vi "execute.vi"(8 "error in (no error)":errorcluster, 9 "B in":refnum<class "GenericComponent.lvclass">, 10 "A in":refnum<class "GenericComponent.lvclass">, 11 "AdapterMH111110ImagingModeToScanHead in":refnum<class "AdapterMH111110ImagingModeToScanHead.lvclass">) -> (0 "error out":errorcluster, 1 "B out":refnum<class "GenericComponent.lvclass">, 2 "A out":refnum<class "GenericComponent.lvclass">, 3 "AdapterMH111110ImagingModeToScanHead out":refnum<class "AdapterMH111110ImagingModeToScanHead.lvclass">)   [LabVIEW 2010, in "AdapterMH111110ImagingModeToScanHead.lvclass"]
uses:
  AdapterMH111110ImagingModeToScanHead.lvclass
  common/classes/GenericComponent/GenericComponent/GenericComponent.lvclass
  ImagingMode/ImagingModeDL090130Frame/ImagingModeDL090130Frame/translation_mode_enum.ctl
  ScanHead/ScanHeadMH100729FPGA/ScanHeadMH100729FPGA/ScanHeadMH100729FPGA.lvclass
  ImagingMode/ImagingModeDL090130Frame/ImagingModeDL090130Frame/settings_cluster.ctl
  ImagingMode/ImagingModeDL090130Frame/ImagingModeDL090130Frame/speed_constant_enum.ctl
  common/xcontrols/XIntensityCompensation/XIntensityCompensation/data.ctl
  ImagingMode/ImagingModeDL090130Frame/ImagingModeDL090130Frame/ImagingModeDL090130Frame.lvclass
  common/xcontrols/XIntensityCompensation/XIntensityCompensation/XIntensityCompensation.xctl
  ScanHead/ScanHeadMH100729FPGA/ScanHeadMH100729FPGA/settings_cluster.ctl
  ScanHead/ScanHeadMH100729FPGA/ScanHeadMH100729FPGA/intensity_adjustment_enum.ctl
  ScanHead/ScanHeadMH100729FPGA/ScanHeadMH100729FPGA/translation_mode_enum.ctl
  common/classes/ErrorController/ErrorController/class_data.vi
  common/classes/ErrorController/ErrorController/ErrorController.lvclass
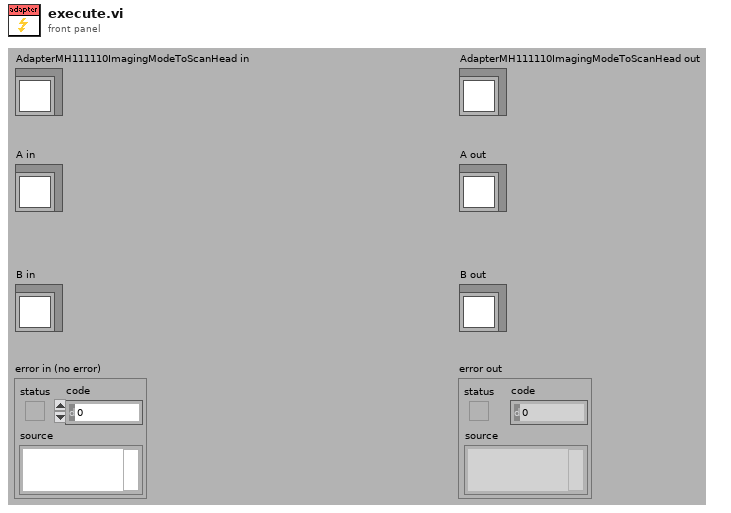
[diagram p1: front panel]
types:
  T1 = typedef "ImagingModeDL090130Frame.lvclass/translation_mode_enum.ctl" = enum16{"scanHead", "stage"}
  T2 = typedef "ImagingModeDL090130Frame.lvclass/settings_cluster.ctl" = cluster{"FrameSettings":cluster{"ResolutionX":i32, "ResolutionY":i32, "AspectRatioX":dbl, "AspectRatioY":dbl, "FrameScanRate":dbl[unit], "SpeedConstant":T3}, "StackSettings":cluster{"Frames":i32, "AveragingRepetitions":i32, "StepSize":dbl[unit], "ReturnToOrigin":bool, "TranslationMode":T1, "IntensityCompensationParameters":T4}}
  T3 = typedef "ImagingModeDL090130Frame.lvclass/speed_constant_enum.ctl" = enum16{"pixel dwell time", "line scan time", "frame rate"}
  T4 = typedef "XIntensityCompensation.xctl/data.ctl" = cluster{"A":dbl, "lambda":dbl[unit], "C":dbl}
  T5 = typedef "ScanHeadMH100729FPGA.lvclass/settings_cluster.ctl" = cluster{"Zoom":dbl, "Intensity":dbl, "AngleZ":dbl[unit], "AngleX":dbl[unit], "OffsetX":dbl[unit], "OffsetY":dbl[unit], "OffsetZ":dbl[unit], "ScatteringLength":dbl[unit], "intensity adjustment mode":T6, "translation mode":T7}
  T6 = typedef "ScanHeadMH100729FPGA.lvclass/intensity_adjustment_enum.ctl" = enum16{"manual", "look-up", "exponential"}
  T7 = typedef "ScanHeadMH100729FPGA.lvclass/translation_mode_enum.ctl" = enum16{"scan signal offset", "stage"}
  T8 = typedef "ImagingModeDL090130Frame.lvclass/control_refs.ctl" = cluster{"resolution controls":cluster{"x pixels":refnum<vi>, "y pixels":refnum<vi>, "ratio x factor":refnum<vi>, "ratio y factor":refnum<vi>}, "speed controls":cluster{"pixel dwell time":refnum<vi>, "line scan time":refnum<vi>, "frame rate":refnum<vi>, "keep constant":refnum<vi>}, "number of frames controls":cluster{"# of frames":refnum<vi>, "duration":refnum<vi>, "# of repetitions":refnum<vi>}, "current value indicators":cluster{"frame #":refnum<vi>, "repetition #":refnum<vi>, "offset":refnum<vi>}, "step controls":cluster{"step size":refnum<vi>, "return to origin?":refnum<vi>, "translation mode":refnum<vi>, "XIntensityCompensation":refnum<vi>}, "defineButton":refnum<vi>, "settings enforced?":refnum<vi>, "settings":refnum<vi>}
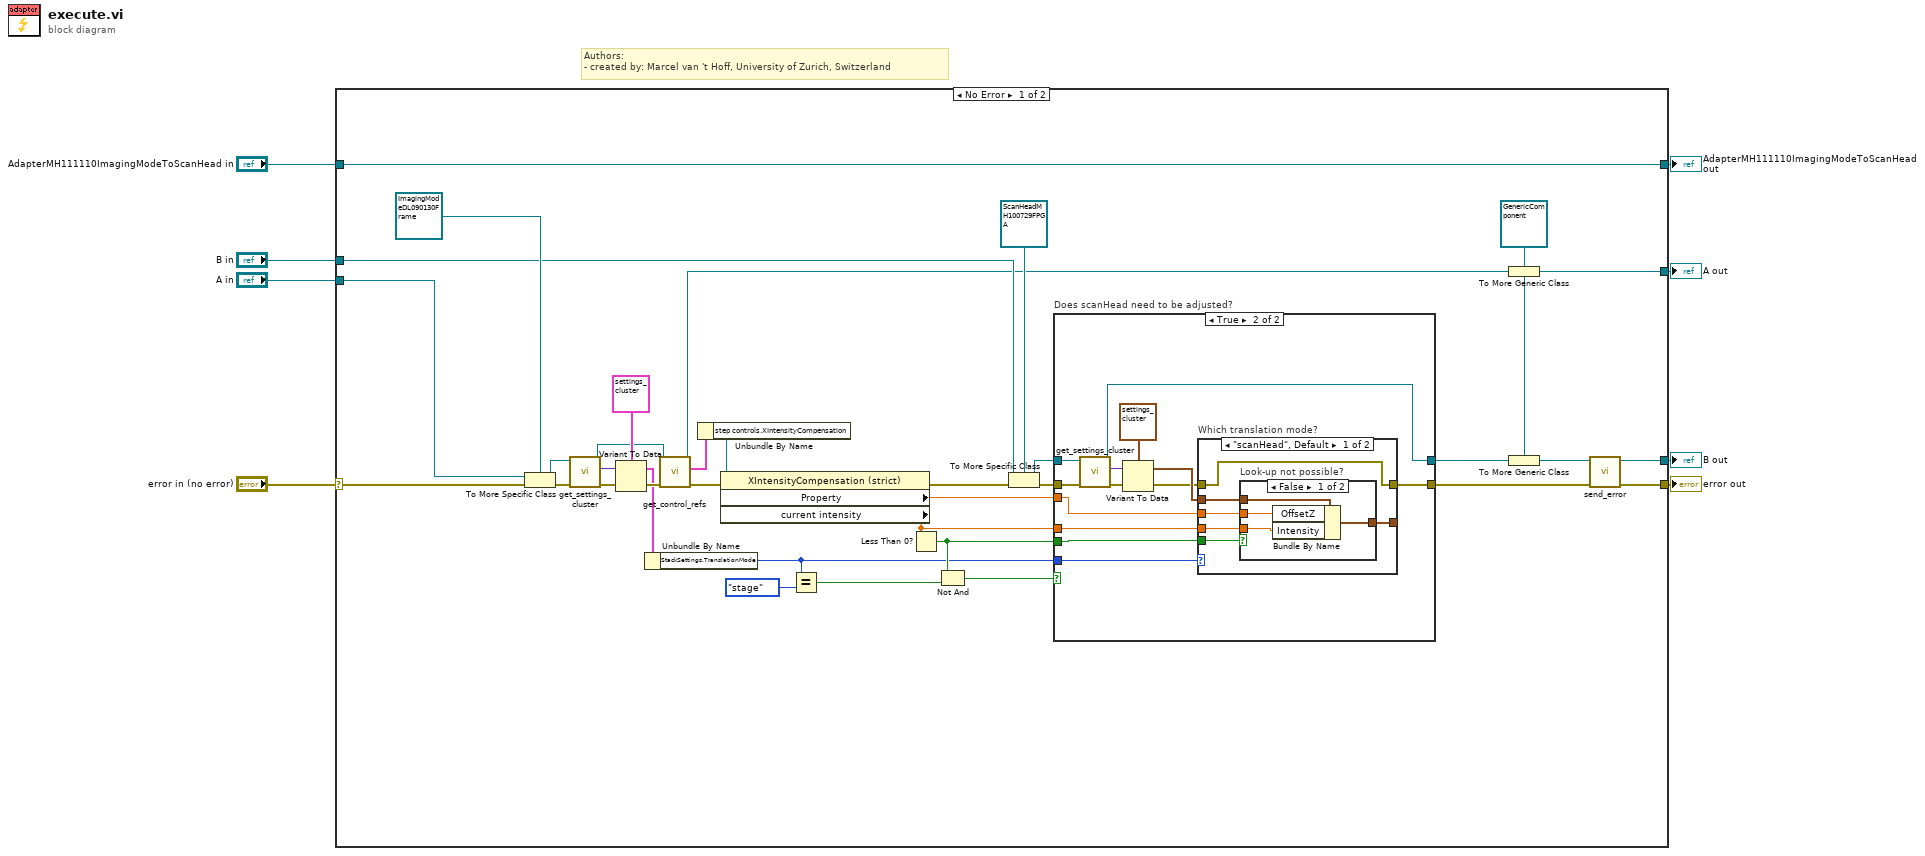
[diagram p0: block diagram]
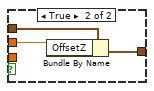
[diagram p3: hidden frame]
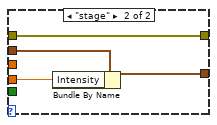
[diagram p4: hidden frame]
diagram:
  # "Authors: \n- created by: Marcel van 't Hoff, University of Zurich, Switzerland"
  n1 = case shown="No Error" "error in (no error)" {
    selector: "error in (no error)" -> [w39 w77]
    tunnel: [w10 w77] -> w7
    tunnel: [w42 w78] -> w6
    tunnel: "AdapterMH111110ImagingModeToScanHead in" -> [w42 w78]
    tunnel: "A in" -> [w41 w75]
    tunnel: "B in" -> [w27 w76]
    tunnel: [w14 w76] -> w2
    tunnel: [w11 w75] -> w1
    frame No Error {
      w13 = refnum<class "GenericComponent.lvclass"> refnum ("GenericComponent.lvclass")
      n2 = To More Specific Class(target class=refnum<class "ImagingModeDL090130Frame.lvclass"> refnum ("ImagingModeDL090130Frame.lvclass"), reference=w41, error in=w39) -> (specific class reference=w37:refnum<class "ImagingModeDL090130Frame.lvclass">, error out=w38:errorcluster)
      n3 = call-dynamic "get_settings_cluster.vi"("error in (no error)"=w38, "ImagingModeDL090130Frame in"=w37) -> ("error out"=w36:errorcluster, "settings cluster"=w35:variant, "ImagingModeDL090130Frame out"=w32:refnum<class "ImagingModeDL090130Frame.lvclass">)  [unwired: 7 in]
      n4 = Variant To Data(error in=w36, Variant=w35, type=T2 {"FrameSettings"={"ResolutionX"=0, "ResolutionY"=0, "AspectRatioX"=0.0, "AspectRatioY"=0.0, "FrameScanRate"=0.0, "SpeedConstant"=enum."pixel dwell time"}, "StackSettings"={"Frames"=0, "AveragingRepetitions"=0, "StepSize"=0.0, "ReturnToOrigin"=FALSE, "TranslationMode"=enum."scanHead", "IntensityCompensationParameters"={"A"=0.0, "lambda"=0.0, "C"=0.0}}} ("settings")) -> (error out=w33:errorcluster, data=w25:T2)
      n5 = Unbundle By Name(w25) -> ("StackSettings.TranslationMode"=w20:T1)
      n6 = call-dynamic "get_control_refs.vi"("error in (no error)"=w33, "ImagingModeDL090130Frame in"=w32) -> ("error out"=w30:errorcluster, "control refs"=w31:T8, "ImagingModeDL090130Frame out"=w12:refnum<class "ImagingModeDL090130Frame.lvclass">)  [unwired: 7 in]
      n7 = Unbundle By Name(w31) -> ("step controls.XIntensityCompensation"=w29:refnum<vi>)
      n8 = property class="XIntensityCompensation (strict)"(reference=w29, error in=w30) -> (error out=w28:errorcluster, "Property"=w19:dbl[unit], "current intensity"=w18:dbl)  [unwired: 1 out]
      n9 = Equal?(x=w20, y=translation_mode_enum."stage") -> (x = y?=w23:bool)
      n10 = Less Than 0?(x=w18) -> (x < 0?=w21:bool)
      n11 = Not And(1:w23, 2:w21) -> (0:w22:bool)
      n12 = To More Specific Class(target class=refnum<class "ScanHeadMH100729FPGA.lvclass"> refnum ("ScanHeadMH100729FPGA.lvclass"), reference=w27, error in=w28) -> (specific class reference=w16:refnum<class "ScanHeadMH100729FPGA.lvclass">, error out=w17:errorcluster)
      n13 = case "Does scanHead need to be adjusted?" shown="True" w22 {
        tunnel: w21 -> [_ w49]
        tunnel: w20 -> [_ w48]
        tunnel: w19 -> [_ w51]
        tunnel: w18 -> [_ w50]
        tunnel: w17 -> [w43 w57]
        tunnel: w16 -> [w44 w56]
        tunnel: [w43 w47] -> w9
        tunnel: [w44 w45] -> w15
        frame False {
        }
        frame True {
          n14 = call-dynamic "get_settings_cluster.vi"("error in (no error)"=w57, "GenericPlugin in"=w56) -> ("error out"=w55:errorcluster, "settings cluster"=w54:variant, "GenericPlugin out"=w45:refnum<class "ScanHeadMH100729FPGA.lvclass">)  [unwired: 7 in]
          n15 = Variant To Data(error in=w55, Variant=w54, type=T5 {"Zoom"=0.0, "Intensity"=0.0, "AngleZ"=0.0, "AngleX"=0.0, "OffsetX"=0.0, "OffsetY"=0.0, "OffsetZ"=0.0, "ScatteringLength"=0.0, "intensity adjustment mode"=enum."manual", "translation mode"=enum."scan signal offset"} ("settings")) -> (error out=w46:errorcluster, data=w52:T5)
          n16 = case "Which translation mode?" shown="\"scanHead\", Default" w48 {
            tunnel: [w63 w72] -> _
            tunnel: w50 -> [w60 w73]
            tunnel: w51 -> [w62 _]
            tunnel: w52 -> [w61 w74]
            tunnel: w49 -> [w59 _]
            tunnel: [w58 w71] -> w47
            tunnel: w46 -> [w58 w71]
            frame "scanHead", Default {
              n17 = case "Look-up not possible?" shown="False" w59 {
                tunnel: [w67 w70] -> w63
                tunnel: w62 -> [w66 w68]
                tunnel: w61 -> [w65 w69]
                tunnel: w60 -> [w64 _]
                frame False {
                  n18 = Bundle By Name(cluster=w65, "OffsetZ"=w66, "Intensity"=w64) -> (w67:T5)
                }
                frame True {
                  n19 = Bundle By Name(cluster=w69, "OffsetZ"=w68) -> (w70:T5)
                }
              }
            }
            frame "stage" {
              n20 = Bundle By Name(cluster=w74, "Intensity"=w73) -> (w72:T5)
            }
          }
        }
      }
      n21 = To More Generic Class(target class=w13, reference=w12) -> (generic class reference=w11:refnum<class "GenericComponent.lvclass">)
      n22 = To More Generic Class(target class=w13, reference=w15) -> (generic class reference=w14:refnum<class "GenericComponent.lvclass">)
      n23 = call "send_error.vi"("error in (no error)"=w9) -> ("error out"=w10:errorcluster)  [unwired: 10 in]
    }
    frame Error {
    }
  }
  "error out" <- w7
  "AdapterMH111110ImagingModeToScanHead out" <- w6
  "A out" <- w1
  "B out" <- w2
